vi "Module Test Example.vi"() -> ()   [LabVIEW 2018, in "Module.lvclass"]
uses:
  Module.lvclass
  support/Message Queue/Message Cluster.ctl
  support/Message Queue/Enqueue Message (Single).vi
  support/Message Queue/Message Queue.lvlib
panel:
  out "Message Queue":refnum<queue>
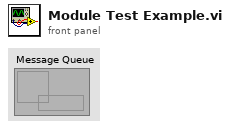
[diagram p1: front panel]
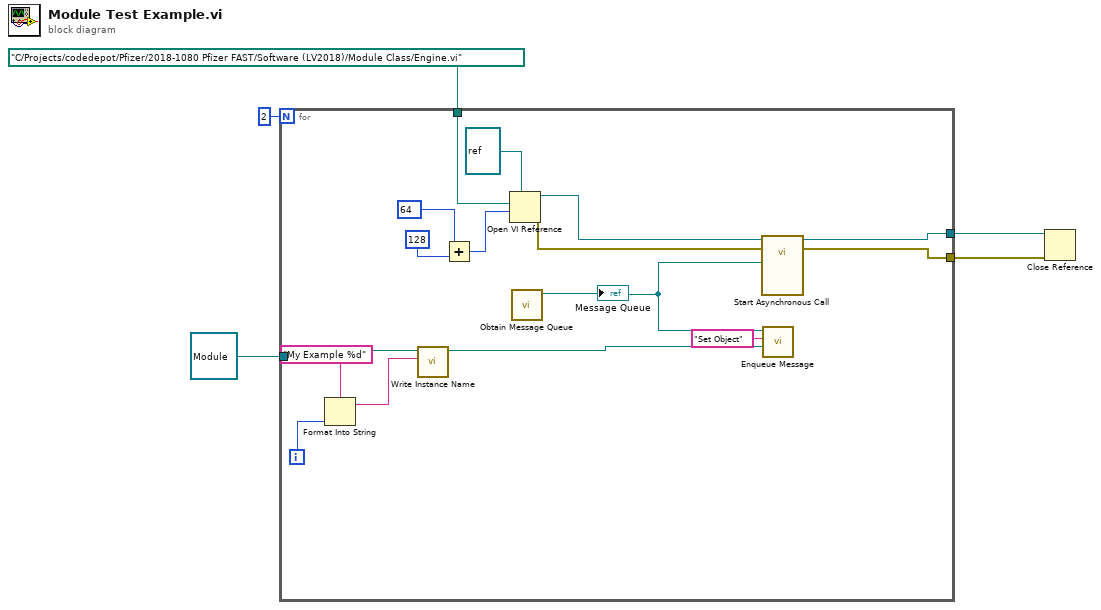
[diagram p0: block diagram]
diagram:
  n1 = for {
    N: 2 -> [_]
    tunnel: path "C:/Projects/codedepot/Pfizer/2018-1080 Pfizer FAST/Software (LV2018)/Module Class/Engine.vi" ("vi path") -> [w21]
    tunnel: refnum<class "Module.lvclass"> refnum ("Module.lvclass") -> [w20]
    tunnel: [w17] -> w3
    tunnel: [w15] -> w2
    i -> [w7]
    n2 = Format Into String(format string="My Example %d" ("Instance Name"), w7) -> (resulting string=w6:string)  [unwired: 2 in, 1 out]
    n3 = call-dynamic "Write Instance Name.vi"("Instance Name"=w6, "Module in"=w20) -> ("Module out"=w13:refnum<class "Module.lvclass">)  [unwired: 8 in, 1 out]
    n4 = Add(x=64 ("options"), y=128 ("options")) -> (x+y=w9:i32)
    n5 = Open VI Reference(type specifier VI Refnum (for type only)=refnum<vi> refnum, vi path=w21, options=w9) -> (vi reference=w18:refnum<vi>, error out=w16:errorcluster)  [unwired: 3 in]
    n6 = call "Obtain Message Queue.vi"() -> ("Message Queue"=w14:refnum<queue>)  [unwired: 10 in, 1 out]
    "Message Queue" <- w14
    n7 = call-by-ref "Start Asynchronous Call"(reference=w18, error in=w16, "Message Queue"=w14) -> (reference out=w17:refnum<vi>, error out=w15:errorcluster)  [unwired: 10 in, 1 out]
    n8 = call-poly "Enqueue Message.vi"("Message Data"=w13, "Message"="Set Object", "Message Queue"=w14) -> ()  [unwired: 7 in, 2 out]
  }
  n9 = Close Reference(reference=w3, error in (no error)=w2) -> ()  [unwired: 1 out]
